vi "Client.vi"() -> ()   [LabVIEW 2016]
doc: "This VI acts as a server for an incoming websockets connection. Receives/sends string data to the connected client.\nWebSockets 1.6.0.22\nSam Sharp - MediaMongrels Ltd\nCopyright (c) 2016, MediaMongrels Ltd"
uses:
  WebSockets/WebSockets.lvlib
panel:
  in  "WS URI":string="ws://localhost:6123/resource/name"
  out "Resource Name":string
  out "Request URI":string
  out "HTTP Headers":variant
  in  "Stop":bool
  out "Received Data":string
  in  "Send":bool
  in  "Data":string
  # "WebSockets Example Client"
  # "This VI is a simple example of sending/receiving data using WebSockets.\nIt waits for a single incoming WebSockets connection on Port 6123 and\nthen displays incoming string data. Strings can also be sent back to the client.\n\nInstructions for use:\n1) Run this VI\n2) Open the index.html file located in the examples folder\n3) The index.html will display the status of the connection and once established, data can be sent/received from either this VI or the index.html file."
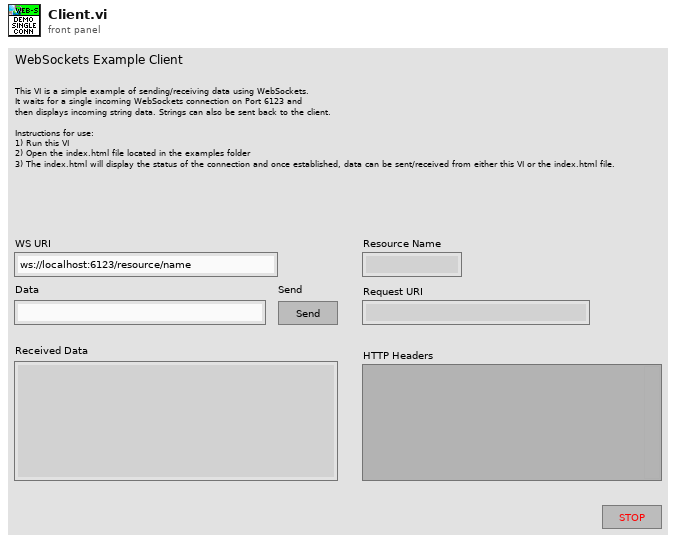
[diagram p1: front panel]
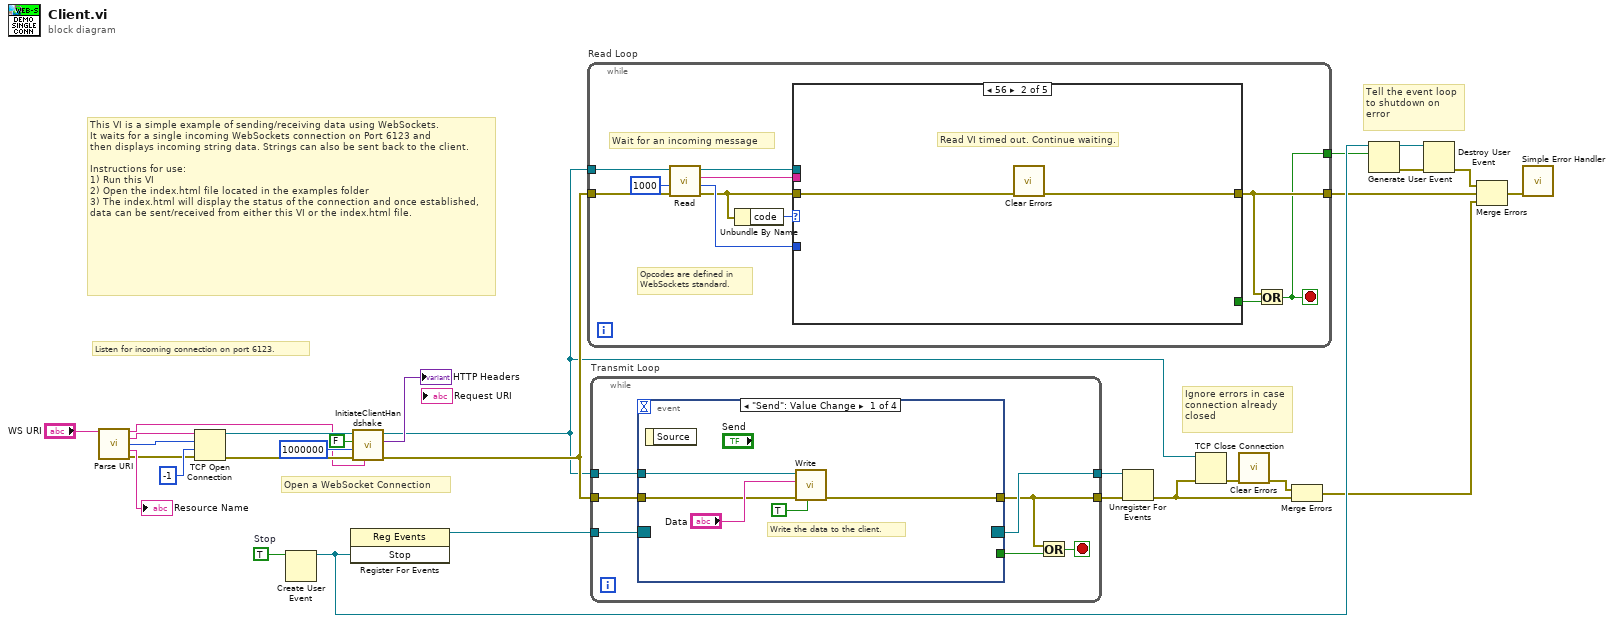
[diagram p0: block diagram]
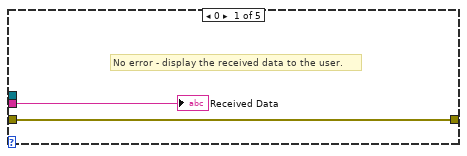
[diagram p2: hidden frame]
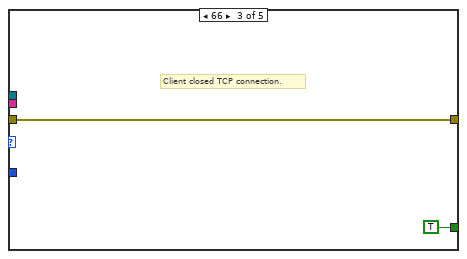
[diagram p3: hidden frame]
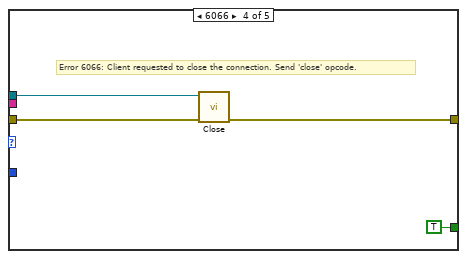
[diagram p4: hidden frame]
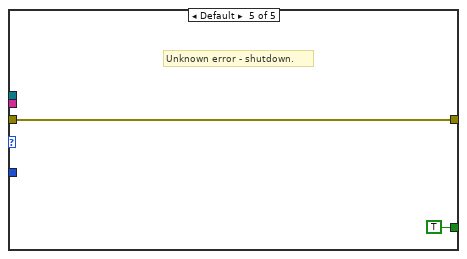
[diagram p5: hidden frame]
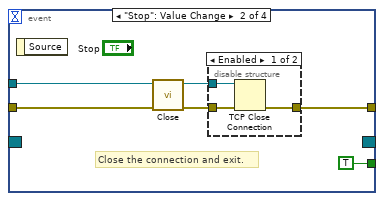
[diagram p6: hidden frame]
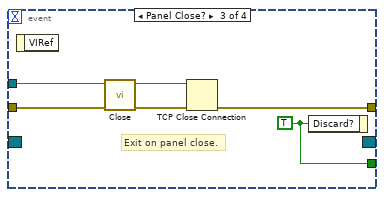
[diagram p8: hidden frame]
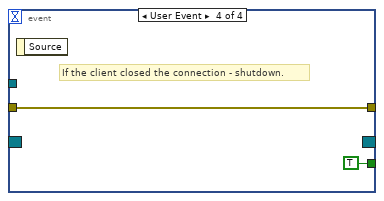
[diagram p9: hidden frame]
diagram:
  w25 = TRUE  # Stop
  # "Ignore errors in case\nconnection already\nclosed"
  # "Tell the event loop to shutdown on error"
  # "This VI is a simple example of sending/receiving data using WebSockets.\nIt waits for a single incoming WebSockets connection on Port 6123 and\nthen displays incoming string data. Strings can also be sent back to the client.\n\nInstructions for use:\n1) Run this VI\n2) Open the index.html file located in the examples folder\n3) The index.html will display the status of the connection and once established, data can be sent/received from either this VI or the index.html file."
  # "Open a WebSocket Connection"
  # "Listen for incoming connection on port 6123."
  n1 = call "Parse URI.vi"("URI"="WS URI") -> ("URI Out"=w6:string, "Hostname"=w5:string, "Port"=w4:u16, "Resource Name"=→"Resource Name":string, "error out"=w2:errorcluster)  [unwired: 9 in, 1 out]
  n2 = TCP Open Connection(address=w5, remote port or service name=w4, timeout ms (60000)=-1 ("timeout ms (25000)"), error in (no error)=w2) -> (connection ID=w28:refnum<k5>, error out=w27:errorcluster)  [unwired: 1 in]
  n3 = Create User Event(user event datatype=w25) -> (user event=w23:refnum<user-event>)  [unwired: 1 in, 1 out]
  n4 = register-events(w23) -> (reference out=w26:refnum<event-registration>)  [unwired: 2 in, 1 out]
  n5 = call "InitiateClientHandshake.vi"("WS URI"=w6, "error in (no error)"=w27, "timeout ms (5000)"=1000000 ("timeout ms (25000)"), "Relative URI Request (F)"=FALSE, "WebSocket Connection in"=w28) -> ("error out"=w14:errorcluster, "Return Headers Out"=→"HTTP Headers":variant, "WebSocket Connection out"=w12:refnum<k5>)  [unwired: 4 in]
  n6 = while "Read Loop" {
    tunnel: w12 -> [w40]
    tunnel: [w30] -> w22
    tunnel: [w32] -> w13
    tunnel: w14 -> [w33]
    stop <- w30 stop-if-true
    # "Wait for an incoming message"
    # "Opcodes are defined in\nWebSockets standard."
    n7 = call "Read.vi"("error in (no error)"=w33, "timeout ms (5000)"=1000 ("timeout ms (25000)"), "WebSocket Connection in"=w40) -> ("error out"=w34:errorcluster, "Opcode"=w35:u8, "Data"=w37:string, "WebSocket Connection out"=w36:refnum<k5>)  [unwired: 5 in]
    n8 = Unbundle By Name(w34) -> ("code"=w38:i32)
    n9 = case shown="56" w38 {
      tunnel: w37 -> [w42 _ _ _ _]
      tunnel: [_ _ TRUE TRUE TRUE] -> w31
      tunnel: w36 -> [_ _ _ w50 _]
      tunnel: w35 -> [_ _ _ _ _]
      tunnel: w34 -> [w41 w44 w45 w48 w51]
      tunnel: [w41 w43 w45 w47 w51] -> w32
      frame 0 {
        # "No error - display the received data to the user."
        "Received Data" <- w42
      }
      frame 56 {
        # "Read VI timed out. Continue waiting."
        n10 = call <vilib>:"Clear Errors.vi"("error in (no error)"=w44) -> ("error out"=w43:errorcluster)  [unwired: 5 in, 1 out]
      }
      frame 66 {
        # "Client closed TCP connection."
      }
      frame 6066 {
        # "Error 6066: Client requested to close the connection. Send 'close' opcode."
        n11 = call "Close.vi"("error in (no error)"=w48, "WebSocket Connection in"=w50) -> ("error out"=w47:errorcluster)  [unwired: 8 in, 1 out]
      }
      frame Default {
        # "Unknown error - shutdown."
      }
    }
    n12 = Or(x=w32, y=w31) -> (x .or. y?=w30:bool)
  }
  n13 = while "Transmit Loop" {
    tunnel: w12 -> [w59]
    tunnel: w26 -> [w58]
    tunnel: [w57] -> w24
    tunnel: [w53] -> w15
    tunnel: w14 -> [w56]
    stop <- w54 stop-if-true
    n14 = event shown="[0] \"Send\": Value Change" {
      selector: w58 -> [_ _ _ _]
      dyn-events: [_ _ _ _] -> w57
      timeout: _ -> [_ _ _ _]
      tunnel: w59 -> [w64 w69 w79 _]
      tunnel: [_ TRUE w77 TRUE] -> w55
      tunnel: [w61 w67 w75 w80] -> w53
      tunnel: w56 -> [w62 w65 w74 w80]
      event "Send": Value Change {
        # "Write the data to the client."
        n15 = event-data() -> ()  [unwired: 1 in, 1 out]
        n16 = call "Write.vi"("Mask payload?"=TRUE, "error in (no error)"=w62, "Data"="Data", "WebSocket Connection in"=w64) -> ("error out"=w61:errorcluster)  [unwired: 6 in, 1 out]
      }
      event "Stop": Value Change {
        # "Close the connection and exit."
        n17 = event-data() -> ()  [unwired: 1 in, 1 out]
        n18 = call "Close.vi"("error in (no error)"=w65, "WebSocket Connection in"=w69) -> ("error out"=w66:errorcluster, "WebSocket Connection in"=w68:refnum<k5>)  [unwired: 8 in]
        n19 = disable-structure shown="Enabled" {
          disable-tunnel: w68 -> [w73 _]
          disable-tunnel: [w72 _] -> w67
          disable-tunnel: w66 -> [w71 _]
          frame Enabled {
            n20 = TCP Close Connection(connection ID=w73, error in (no error)=w71) -> (error out=w72:errorcluster)  [unwired: 1 in, 1 out]
          }
          frame Disabled {
          }
        }
      }
      event Panel Close? {
        w77 = TRUE ("Discard?")
        # "Exit on panel close."
        n21 = event-data() -> ()  [unwired: 1 in, 1 out]
        n22 = call "Close.vi"("error in (no error)"=w74, "WebSocket Connection in"=w79) -> ("error out"=w76:errorcluster, "WebSocket Connection in"=w78:refnum<k5>)  [unwired: 8 in]
        n23 = TCP Close Connection(connection ID=w78, error in (no error)=w76) -> (error out=w75:errorcluster)  [unwired: 1 in, 1 out]
        n24 = event-data("Discard?"=w77) -> ()  [unwired: 1 in, 1 out]
      }
      event User Event {
        # "If the client closed the connection - shutdown."
        n25 = event-data() -> ()  [unwired: 1 in, 1 out]
      }
    }
    n26 = Or(x=w53, y=w55) -> (x .or. y?=w54:bool)
  }
  n27 = Unregister For Events(event registration refnum=w24, error in=w15) -> (error out=w10:errorcluster)
  n28 = TCP Close Connection(connection ID=w12, error in (no error)=w10) -> (error out=w11:errorcluster)  [unwired: 1 in, 1 out]
  n29 = call <vilib>:"Clear Errors.vi"("error in (no error)"=w11) -> ("error out"=w8:errorcluster)  [unwired: 5 in, 1 out]
  n30 = Merge Errors(w8, w10) -> (w9:errorcluster)
  n31 = Generate User Event(user event=w23, event data cluster=w22) -> (user event out=w21:refnum<user-event>, error out=w20:errorcluster)  [unwired: 2 in]
  n32 = Destroy User Event(user event=w21, error in=w20) -> (error out=w19:errorcluster)
  n33 = Merge Errors(w19, w13, w9) -> (w16:errorcluster)
  n34 = call <vilib>:"Simple Error Handler.vi"("error in (no error)"=w16) -> ()  [unwired: 4 in, 5 out]
